vi "controlFrequency.vi"(7 "Set":bool, 8 "error in":errorcluster, 9 "Frequenzy [Hz] in":dbl, 10 "axis in":u8, 11 "connection ID":refnum<k5>) -> (0 "error out":errorcluster, 1 "Frequenzy [Hz] out":dbl, 2 "axis out":u8, 3 "connection ID":refnum<k5>)   [LabVIEW 2016]
doc: "This function retrieves or sets the frequency of the actuator signal of the selected axis."
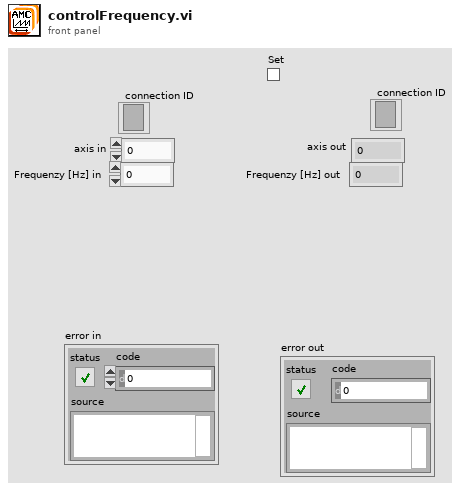
[diagram p1: front panel]
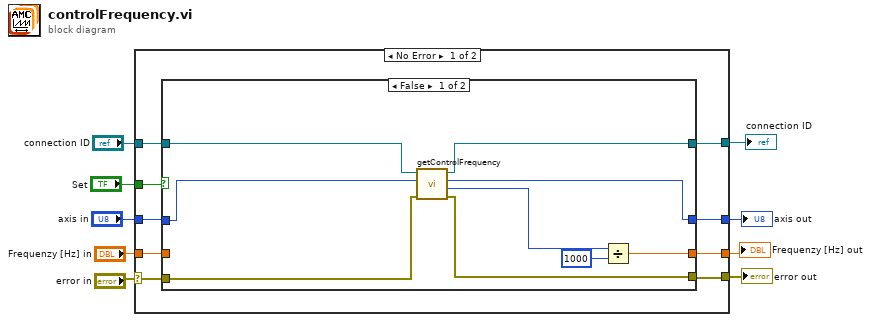
[diagram p0: block diagram]
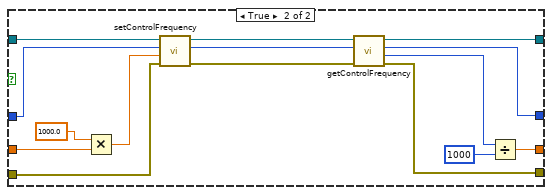
[diagram p2: hidden frame]
diagram:
  n1 = case shown="No Error" "error in" {
    selector: "error in" -> [w14 w46]
    tunnel: "axis in" -> [w16 w44]
    tunnel: [w10 w46] -> w8
    tunnel: [w12 w44] -> w7
    tunnel: "Frequenzy [Hz] in" -> [w15 w45]
    tunnel: [w11 w45] -> w5
    tunnel: "Set" -> [w17 _]
    tunnel: [w13 w43] -> w3
    tunnel: "connection ID" -> [w18 w43]
    frame No Error {
      n2 = case shown="False" w17 {
        tunnel: [w26 w36] -> w13
        tunnel: w18 -> [w27 w42]
        tunnel: w16 -> [w24 w30]
        tunnel: [w20 w28] -> w12
        tunnel: [w25 w33] -> w10
        tunnel: [w21 w31] -> w11
        tunnel: w15 -> [_ w40]
        tunnel: w14 -> [w19 w38]
        frame False {
          n3 = call "getControlFrequency.vi"("error in"=w19, "axis"=w24, "connection ID"=w27) -> ("error out"=w25:errorcluster, "frequency"=w23:i32, "axis_out"=w20:i32, "connection ID"=w26:refnum<k5>)  [unwired: 5 in]
          n4 = Divide(x=w23, y=1000) -> (x/y=w21:dbl)
        }
        frame True {
          n5 = Multiply(x=1000.0, y=w40) -> (x*y=w39:dbl)
          n6 = call "setControlFrequency.vi"("error in"=w38, "frequency"=w39, "axis"=w30, "connection ID"=w42) -> ("error out"=w34:errorcluster, "axis_out"=w29:i32, "connection ID"=w37:refnum<k5>)  [unwired: 5 in]
          n7 = call "getControlFrequency.vi"("error in"=w34, "axis"=w29, "connection ID"=w37) -> ("error out"=w33:errorcluster, "frequency"=w32:i32, "axis_out"=w28:i32, "connection ID"=w36:refnum<k5>)  [unwired: 5 in]
          n8 = Divide(x=w32, y=1000) -> (x/y=w31:dbl)
        }
      }
    }
    frame Error {
    }
  }
  "error out" <- w8
  "axis out" <- w7
  "Frequenzy [Hz] out" <- w5
  "connection ID" <- w3
